vi "Split and Format Tables.vi"(0 "Header":string[](array[string]), 5 "Data Table":dbl[][](array[numeric]), 7 "End Index":i32=1) -> (4 "spreadsheet string":string)   [LabVIEW 2010]
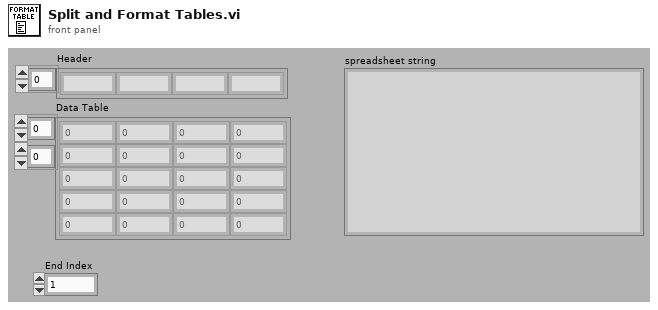
[diagram p1: front panel]
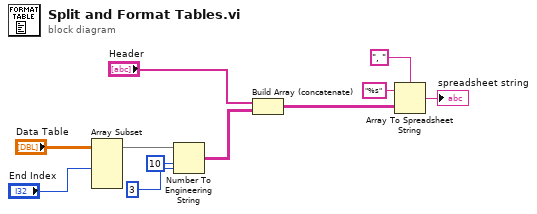
[diagram p0: block diagram]
diagram:
  n1 = Array Subset(array="Data Table", length (row)="End Index") -> (w2:dbl[][])  [unwired: 3 in]
  n2 = Number To Engineering String(2:i16 3 ("precision (6)"), 3:i16 10 ("width (-)"), 4:w2) -> (0:w9:string[][])  [unwired: 1 in]
  n3 = Build Array (concatenate)("Header", w9) -> (w7:string[][])
  n4 = Array To Spreadsheet String(delimiter (Tab)=", ", array=w7, 3:"%s" ("format string")) -> (spreadsheet string=→"spreadsheet string":string)
